vi "Main_SAIDD_1while.vi"() -> ()   [LabVIEW 2018]
uses:
  <vilib>/myRIO/Common/Instrument Driver Framework/myRIO v1.0/UART/vis/myRIO v1.0 Close UART.vi
  <vilib>/Utility/error.llb/Error Cluster From Error Code.vi
  <vilib>/myRIO/Common/Instrument Driver Framework/myRIO v1.0/PWM/vis/myRIO v1.0 Write PWM.vi
  <vilib>/myRIO/Common/Instrument Driver Framework/myRIO v1.0/DIO/vis/myRIO v1.0 Write DIO.vi
  <vilib>/myRIO/Common/Instrument Driver Framework/Utilities/vis/FPGA Ref Manager.vi
  <vilib>/myRIO/Common/Instrument Driver Framework/myRIO v1.0/myRIO v1.0 Reset FPGA.vi
  <vilib>/myRIO/Common/Instrument Driver Framework/myRIO v1.0/IRQ/vis/myRIO v1.0 IRQ Info FGV.vi
  <vilib>/myRIO/Common/Instrument Driver Framework/myRIO v1.0/IRQ/vis/myRIO v1.0 Timer IRQ Info FGV.vi
  <vilib>/myRIO/Common/Instrument Driver Framework/myRIO v1.0/IRQ/vis/myRIO v1.0 ISR Agent.vi
  <vilib>/myRIO/Instrument Drivers/Onboard IO/DIO/DIO.lvlib
  <vilib>/myRIO/Instrument Drivers/Onboard IO/PWM/PWM.lvlib
  <vilib>/myRIO/Instrument Drivers/Utilities/Utilities.lvlib
panel:
  in  "Filter?":bool=TRUE
  out "RollDetection - Alarm":bool
  in  "Radius":dbl=0.005 format="%#_13g"
  in  "high cutoff freq:":dbl=900.0
  in  "Grounded threshold":dbl=1.7 format="%#_13g"
  in  "Enable Triangle Wobble":bool=TRUE
  in  "Antal iterationer pr. stepper":i32=800
  in  "Stop":bool
  out "Measured current":dbl
  out "Ammeter measurement":dbl(graph)
  out "Duty Cycle":dbl
  out "Mean 200":dbl format="%0.2f"
  out "Battery left (%)":dbl
  in  "Drill - Frequency [Hz]":dbl=200.0
  in  "Stepper frekvens ned":dbl=120.0
  in  "Ingen modstand ned upper threshold":dbl=2750.0
  out "ALL TOP":bool
  out "ALL BOTTOM":bool
  in  "Resistance - Threshold Upper":dbl=3100.0
  in  "Resistance Threshold Lower":dbl=3025.0
  out "Process":T1(ring)
  in  "State":T1(ring)
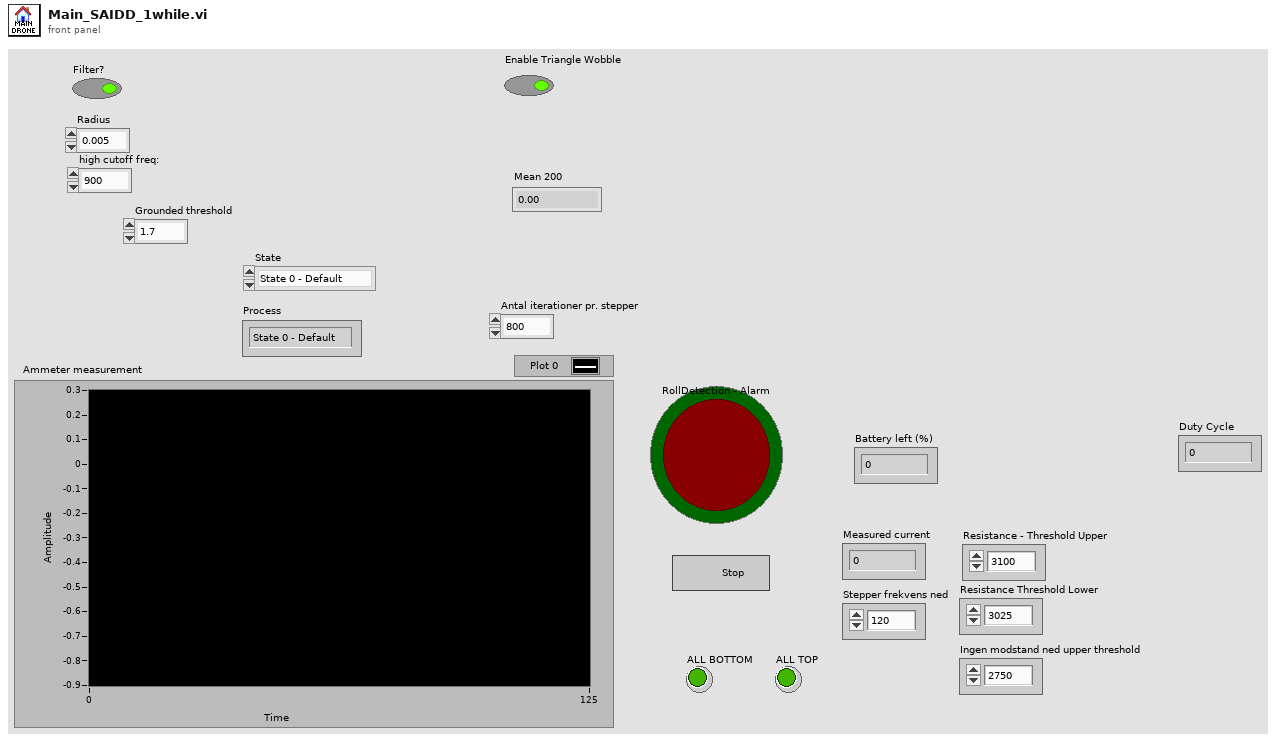
[diagram p1: front panel]
types:
  T1 = enum16{"State 0 - Default", "State 1 - Go down", "State 2 - Go up", "State 3 - Triangle Wobble"}
  T2 = typedef "DIO.lvlib/DIO Reference.ctl" = cluster{"myRIO Reference":T3, "DIO Channels List":T7}
  T3 = typedef "myRIO Generic Hardware Reference.ctl" = cluster{"myRIO Model":T4, "myRIO Hardware Reference":T5}
  T4 = typedef "Hardware Version Enum.ctl" = enum16{"Unknown", "myRIO-1900", "myRIO-1950", "roboRIO", "NI ELVIS RIO CM", "ELVIS III"}
  T5 = typedef "myRIO v1.0 Reference.ctl" = cluster{"Generic FPGA Reference":T6, "Allow multiple opens":bool}
  T6 = typedef "Generic FPGA Reference.ctl" = refnum<k20>
  T7 = typedef "DIO Channels List.ctl" = T8[]
  T8 = typedef "DIO Channels Enum.ctl" = enum16{"Not Connected", "C/DIO0", "C/DIO1", "C/DIO2", "C/DIO3", "C/DIO4", "C/DIO5", "C/DIO6", "C/DIO7", "A/DIO0", "A/DIO1", "A/DIO2", "A/DIO3", "A/DIO4", "A/DIO5", "A/DIO6", "A/DIO7", "A/DIO8", "A/DIO9", "A/DIO10", "A/DIO11", "A/DIO12", "A/DIO13", "A/DIO14", "A/DIO15", "A/DIO16", "A/DIO17", "A/DIO18", "A/DIO19", "B/DIO0", "B/DIO1", "B/DIO2", "B/DIO3", "B/DIO4", "B/DIO5", "B/DIO6", "B/DIO7", "B/DIO8", "B/DIO9", "B/DIO10", "B/DIO11", "B/DIO12", "B/DIO13", "B/DIO14", "B/DIO15", "B/DIO16", "B/DIO17", "B/DIO18", "B/DIO19", "LED0", "LED1", "LED2", "LED3", "Button0", "DIO/DIO0", "DIO/DIO1", "DIO/DIO2", "DIO/DIO3", "DIO/DIO4", "DIO/DIO5", "DIO/DIO6", "DIO/DIO7", "DIO/DIO8", "DIO/DIO9", "SPI/CS0", "SPI/CS1", "SPI/CS2", "SPI/CS3", "LED RADIO (Green)", "LED RADIO (Red)", "LED COMM (Green)", "LED COMM (Red)", "LED MODE (Green)", "LED MODE (Red)"}
  T9 = typedef "PWM.lvlib/PWM Reference.ctl" = cluster{"myRIO Reference":T3, "PWM Channels Enum":T10, "PWM Configuration":T11}
  T10 = typedef "PWM Channels Enum.ctl" = enum16{"Not Connected", "C/PWM0", "C/PWM1", "A/PWM0", "A/PWM1", "A/PWM2", "A/PWM3", "A/PWM4", "A/PWM5", "A/PWM6", "A/PWM7", "A/PWM8", "A/PWM9", "A/PWM10", "A/PWM11", "A/PWM12", "A/PWM13", "A/PWM14", "A/PWM15", "A/PWM16", "A/PWM17", "A/PWM18", "A/PWM19", "B/PWM0", "B/PWM1", "B/PWM2", "B/PWM3", "B/PWM4", "B/PWM5", "B/PWM6", "B/PWM7", "B/PWM8", "B/PWM9", "B/PWM10", "B/PWM11", "B/PWM12", "B/PWM13", "B/PWM14", "B/PWM15", "B/PWM16", "B/PWM17", "B/PWM18", "B/PWM19", "PWM/PWM0", "PWM/PWM1", "PWM/PWM2", "PWM/PWM3", "PWM/PWM4", "PWM/PWM5", "PWM/PWM6", "PWM/PWM7", "PWM/PWM8", "PWM/PWM9"}
  T11 = typedef "PWM.lvlib/PWM Configuration.ctl" = cluster{"Frequency":dbl, "Duty Cycle":dbl}
  T12 = typedef "Accelerometer.lvlib/Accelerometer Reference.ctl" = cluster{"myRIO Reference":T3, "Accelerometer Channels List":T13, "LSB Weight":dbl}
  T13 = typedef "Accelerometer Channels List.ctl" = T14[]
  T14 = typedef "Accelerometer Channels Enum.ctl" = enum16{"Not Connected", "X-Axis", "Y-Axis", "Z-Axis"}
  T15 = typedef "AI.lvlib/AI Reference.ctl" = cluster{"myRIO Reference":T3, "AI Channels List":T16, "AI Scaling Constants List":T18}
  T16 = typedef "AI Channels List.ctl" = T17[]
  T17 = typedef "AI Channels Enum.ctl" = enum16{"Not Connected", "AudioIn/Left", "AudioIn/Right", "C/AI0", "C/AI1", "A/AI0", "A/AI1", "A/AI2", "A/AI3", "A/AI4", "A/AI5", "A/AI6", "A/AI7", "B/AI0", "B/AI1", "B/AI2", "B/AI3", "B/AI4", "B/AI5", "B/AI6", "B/AI7", "AI/AI0", "AI/AI1", "AI/AI2", "AI/AI3", "A/AI0 (DIFF)", "A/AI1 (DIFF)", "A/AI2 (DIFF)", "A/AI3 (DIFF)", "B/AI0 (DIFF)", "B/AI1 (DIFF)", "B/AI2 (DIFF)", "B/AI3 (DIFF)"}
  T18 = typedef "Analog Scaling Constants List.ctl" = T19[]
  T19 = typedef "Analog Scaling Constants.ctl" = cluster{"LSB Weight (Volts)":dbl, "Offset (Volts)":dbl, "Signed?":bool}
  T20 = typedef "SPI.lvlib/SPI Reference.ctl" = cluster{"myRIO Reference":T3, "SPI Channels Enum":T21, "SPI Configuration":T22}
  T21 = typedef "SPI Channels Enum.ctl" = enum16{"Not Connected", "A/SPI", "B/SPI", "SPI/SPI"}
  T22 = typedef "SPI.lvlib/SPI Configuration.ctl" = cluster{"Frequency [Hz]":dbl, "Clock Phase":T23, "Clock Polarity":T24, "Data Direction":T25, "Frame Length":T26}
  T23 = typedef "SPI Clock Phase.ctl" = enum8{"Leading", "Trailing"}
  T24 = typedef "SPI Clock Polarity.ctl" = enum8{"Low", "High"}
  T25 = typedef "SPI Data Direction.ctl" = enum8{"Most significant bit first", "Least significant bit first"}
  T26 = typedef "SPI Frame Length.ctl" = u8
  T27 = cluster{"B/DIO0 - Stepper Direction":T2, "B/DIO1 - Stepper1 Enable":T2, "B/DIO2 - Stepper2 Enable":T2, "B/DIO3 - Stepper3 Enable":T2, "B/DIO4 - Endstop Stepper1 Top":T2, "B/DIO11 - Endstop Stepper1 Bund":T2, "B/DIO12 - Endstop Stepper2 Top":T2, "B/DIO13 - Endstop Stepper2 Bund":T2, "B/DIO14 - Endstop Stepper3 Top":T2, "B/DIO15 - Endstop Stepper3 Bund":T2, "Deleted - A/DIO0 - Cooler":T2, "A/DIO1 - Beacon drop (dio1)":T2, "A/DIO2 - Beacon drop (dio0)":T2, "A/DIO3 - QuickRelease (dio1)":T2, "A/DIO4 - QuickRelease (dio0)":T2, "Deleted - A/DIO11 - LiDAR SPI CS":T2, "B/PWM0 - Stepper":T9, "B/PWM1 - Drill":T9, "Deleted - A/PWM0 - Servo_Roll":T9, "Deleted - A/PWM1 - Servo_Yaw":T9, "Acc. X-axis":T12, "Acc. Y-axis":T12, "B/AI0 - Drone Grounded S1 - F3":T15, "A/AI0 - QuickRelease S4 - F4":T15, "B/AI2 - Beacon Drop S5 - F5":T15, "B/AI3 - Begin drilling S3 - F6":T15, "B/AI1 - Gimbal Seach S8 - F8":T15, "Deleted - A/AI1 - Beacon Wiper":T15, "A/AI2 - QuickRelease Wiper":T15, "A/AI3 - Drill Current":T15, "Deleted - A/SPI - LiDAR":T20, "B/UART - XBee":refnum<visa-resource-name>, "Deleted - A/UART - A3 GPS":refnum<visa-resource-name>, "RIO Flashing LEDs":T2}
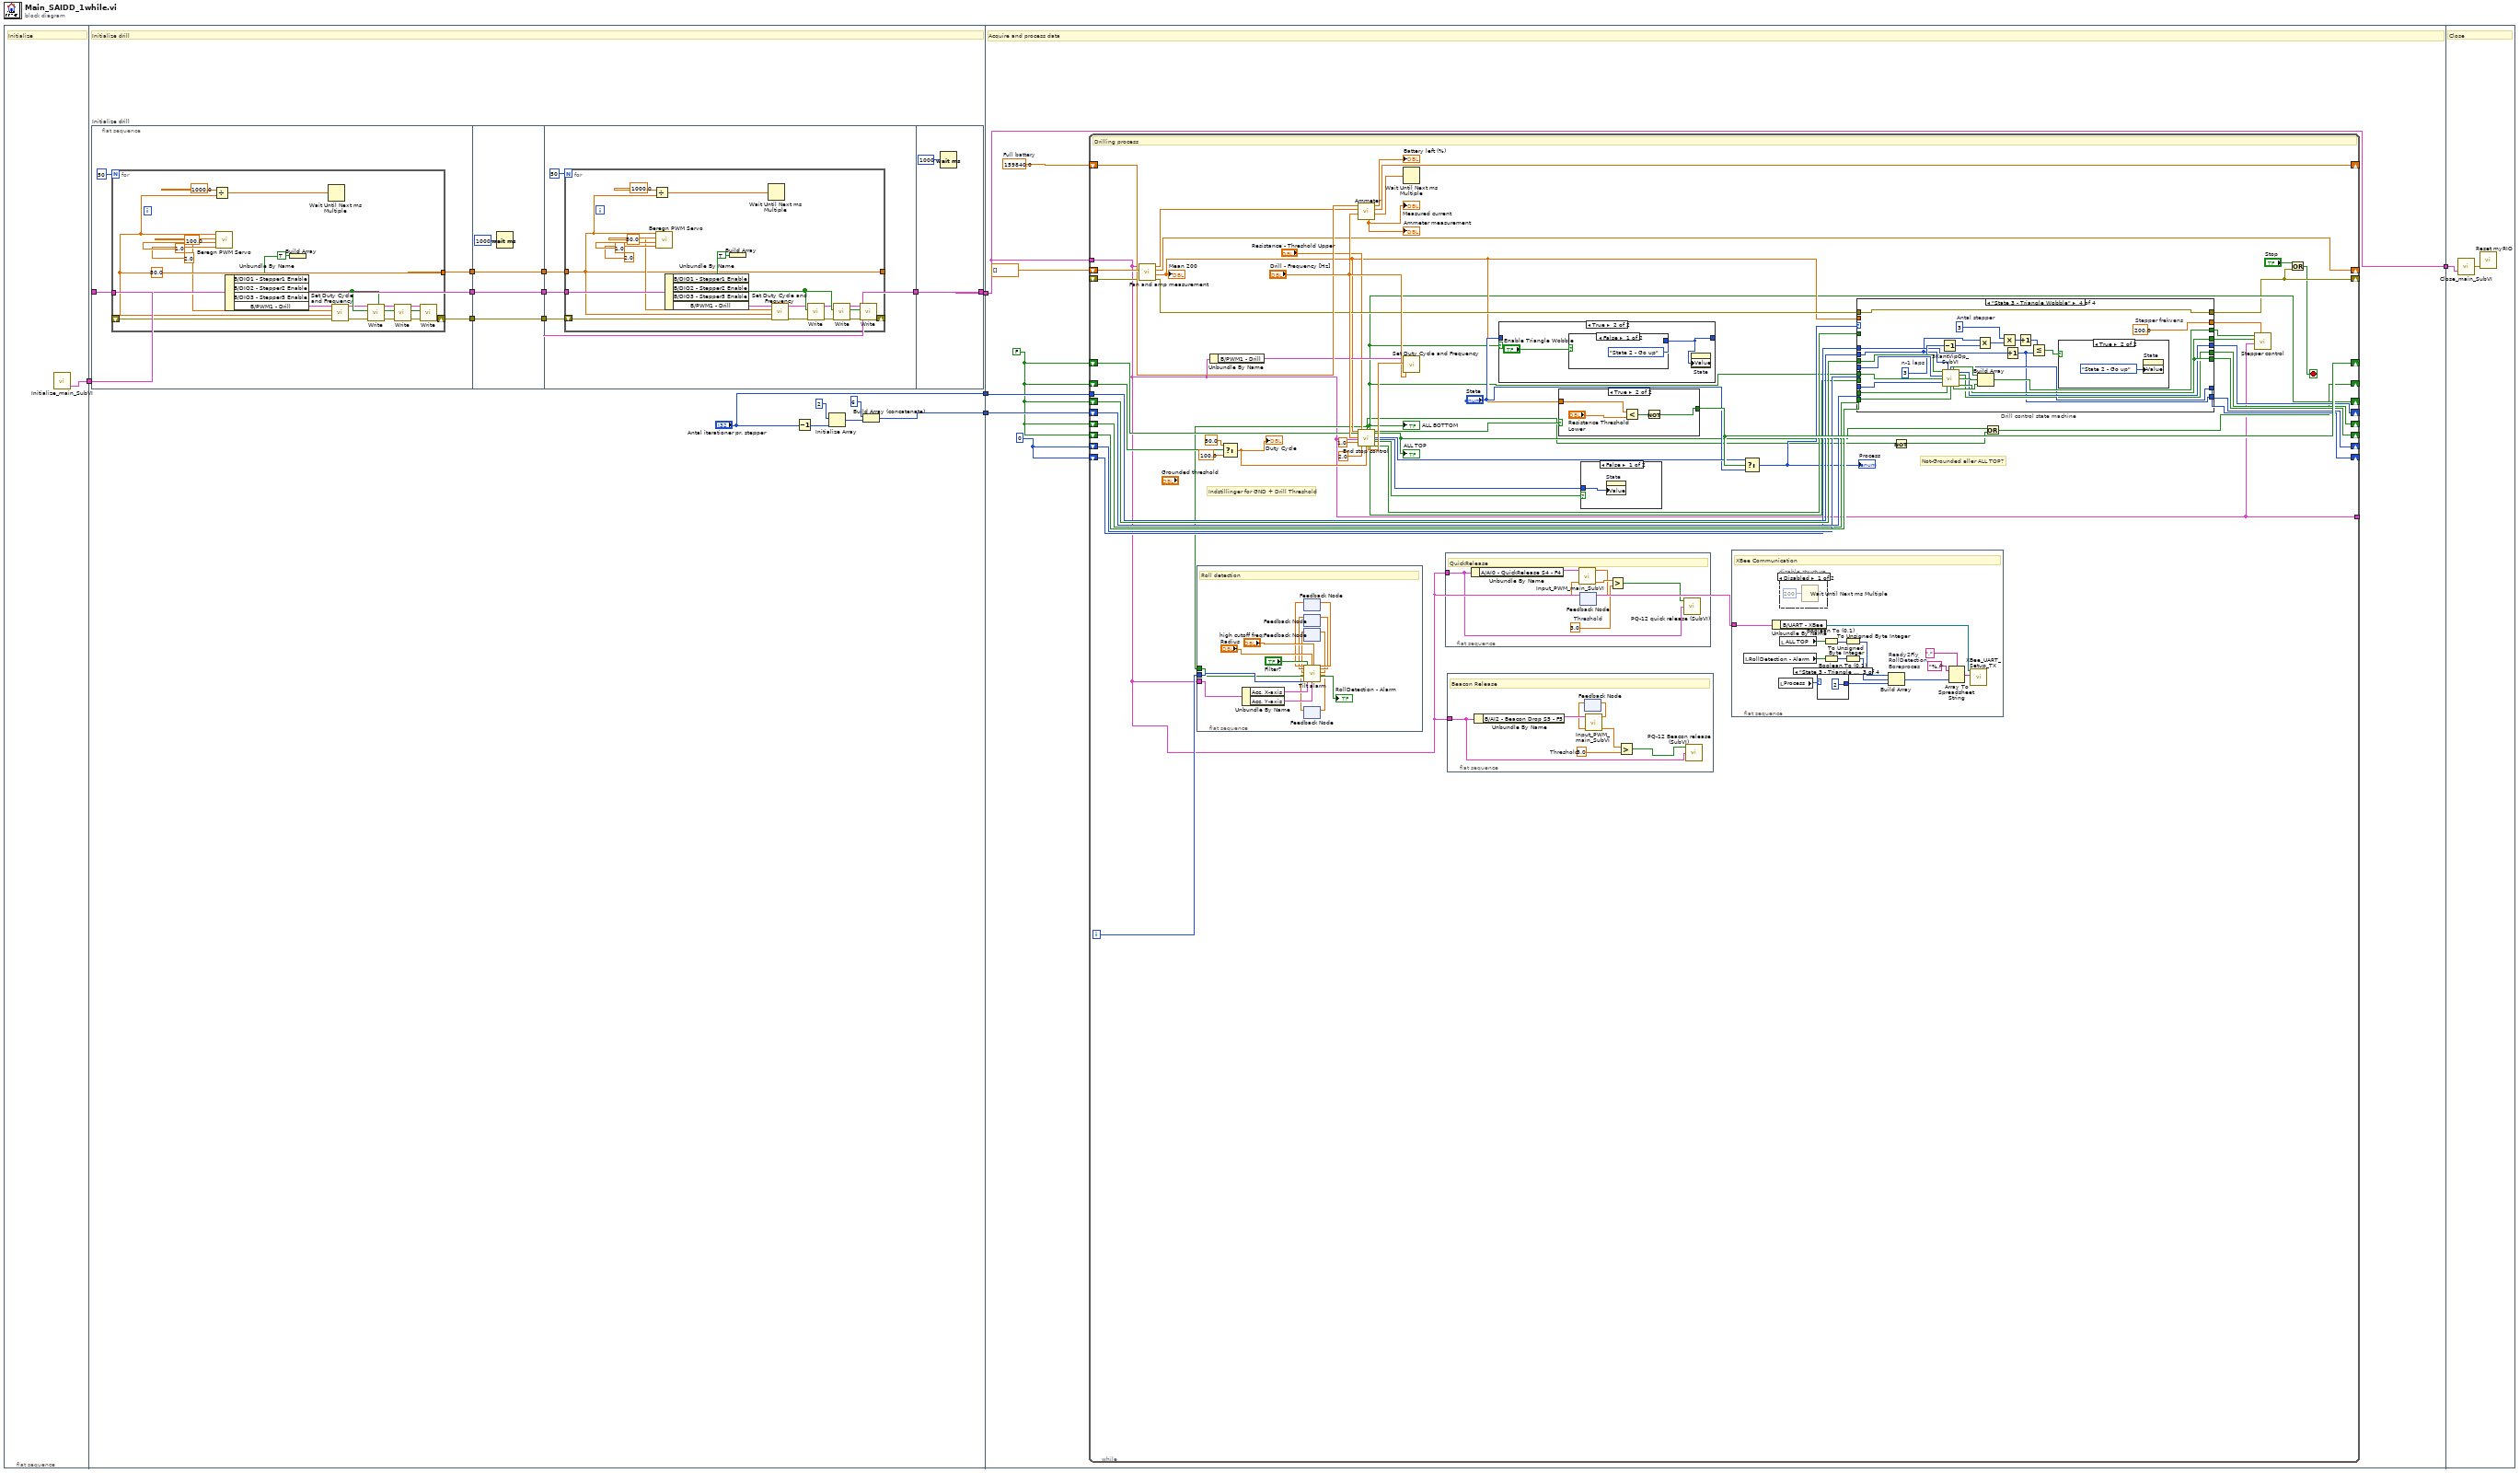
[diagram p0: block diagram]
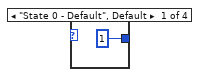
[diagram p3: hidden frame]
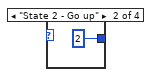
[diagram p4: hidden frame]
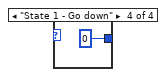
[diagram p5: hidden frame]
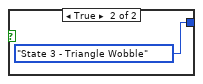
[diagram p8: hidden frame]
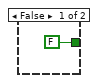
[diagram p9: hidden frame]
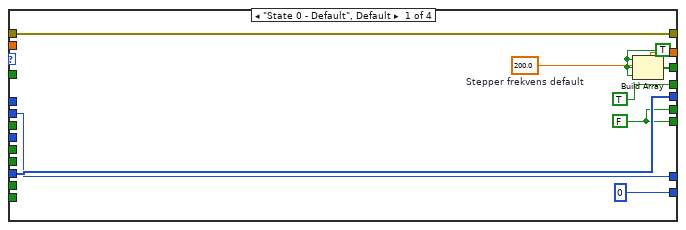
[diagram p10: hidden frame]
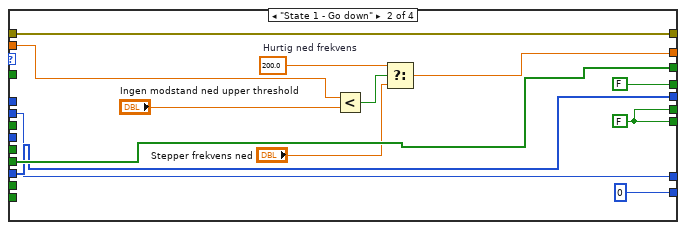
[diagram p11: hidden frame]
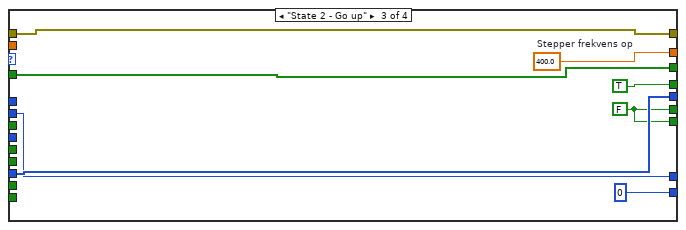
[diagram p12: hidden frame]
diagram:
  n1 = flat-sequence {
    tunnel: [w6] -> w4
    tunnel: w4 -> [w21]
    tunnel: [w18] -> w3
    tunnel: ["Antal iterationer pr. stepper"] -> w2
    tunnel: [w12] -> w1
    tunnel: w3 -> [w74]
    tunnel: [w74] -> w5
    tunnel: w2 -> [w77]
    tunnel: w1 -> [w76]
    tunnel: w5 -> [w256]
    frame #0 {
      # "Initialize"
      n2 = call "Initialize_main_SubVI.vi"() -> ("output cluster"=w6:T27)  [unwired: 2 in, 1 out]
    }
    frame #1 {
      # "Initialize drill"
      n3 = flat-sequence "Initialize drill" {
        tunnel: w21 -> [w25]
        tunnel: [w25] -> w20
        tunnel: [w24] -> w9
        tunnel: [w23] -> w7
        tunnel: w20 -> [w48]
        tunnel: [w48] -> w19
        tunnel: [w46] -> w10
        tunnel: w9 -> [w46]
        tunnel: [w45] -> w8
        tunnel: w7 -> [w45]
        tunnel: w19 -> [w52]
        tunnel: [w52] -> w17
        tunnel: w10 -> [w51]
        tunnel: w8 -> [w50]
        tunnel: [w73] -> w18
        tunnel: w17 -> [w73]
        frame #0 {
          n4 = for {
            N: 50 -> [_]
            tunnel: [w39] -> w24
            shift-right: [w32] -> w23
            shift-left: _ -> [w41]
            tunnel: w25 -> [w37]
            w39 = 50.0 ("Frequency [Hz]")
            n5 = Divide(x=1000.0, y=w39) -> (x/y=w40:dbl)
            n6 = call "Beregn PWM Servo.vi"("Max (ms puls bredde)"=2.0, "Min (ms puls bredde)"=1.0, "Duty Cycle"=100.0, "Frekvens"=w39) -> ("Output Dutycycle til PWM Servo"=w26:dbl)  [unwired: 7 in]
            n7 = Unbundle By Name(w37) -> ("B/DIO1 - Stepper1 Enable"=w27:T2, "B/DIO2 - Stepper2 Enable"=w28:T2, "B/DIO3 - Stepper3 Enable"=w29:T2, "B/PWM1 - Drill"=w31:T9)
            n8 = Build Array(TRUE) -> (w30:bool[])
            n9 = Wait Until Next ms Multiple(millisecond multiple=w40) -> ()  [unwired: 1 out]
            n10 = call <vilib>:"Set Duty Cycle and Frequency.vi"("error in (no error)"=w41, "Frequency [Hz]"=w39, "Duty Cycle"=w26, "PWM Ref In"=w31) -> ("error out"=w35:errorcluster)  [unwired: 5 in, 1 out]
            n11 = call <vilib>:"Write.vi"("error in (no error)"=w35, "Values"=w30, "DIO Ref In"=w29) -> ("error out"=w34:errorcluster)  [unwired: 6 in, 1 out]
            n12 = call <vilib>:"Write.vi"("error in (no error)"=w34, "Values"=w30, "DIO Ref In"=w28) -> ("error out"=w33:errorcluster)  [unwired: 6 in, 1 out]
            n13 = call <vilib>:"Write.vi"("error in (no error)"=w33, "Values"=w30, "DIO Ref In"=w27) -> ("error out"=w32:errorcluster)  [unwired: 6 in, 1 out]
          }
        }
        frame #1 {
          n14 = Wait (ms)(milliseconds to wait=u32 1000) -> ()  [unwired: 1 out]
        }
        frame #2 {
          n15 = for {
            N: 50 -> [_]
            tunnel: [w53] -> _
            shift-right: [w60] -> _
            shift-left: w50 -> [w68]
            tunnel: w52 -> [w65]
            tunnel: w51 -> [w53]
            n16 = Divide(x=1000.0, y=w53) -> (x/y=w67:dbl)
            n17 = call "Beregn PWM Servo.vi"("Max (ms puls bredde)"=2.0, "Min (ms puls bredde)"=1.0, "Duty Cycle"=50.0, "Frekvens"=w53) -> ("Output Dutycycle til PWM Servo"=w54:dbl)  [unwired: 7 in]
            n18 = Unbundle By Name(w65) -> ("B/DIO1 - Stepper1 Enable"=w55:T2, "B/DIO2 - Stepper2 Enable"=w56:T2, "B/DIO3 - Stepper3 Enable"=w57:T2, "B/PWM1 - Drill"=w59:T9)
            n19 = Build Array(TRUE) -> (w58:bool[])
            n20 = Wait Until Next ms Multiple(millisecond multiple=w67) -> ()  [unwired: 1 out]
            n21 = call <vilib>:"Set Duty Cycle and Frequency.vi"("error in (no error)"=w68, "Frequency [Hz]"=w53, "Duty Cycle"=w54, "PWM Ref In"=w59) -> ("error out"=w63:errorcluster)  [unwired: 5 in, 1 out]
            n22 = call <vilib>:"Write.vi"("error in (no error)"=w63, "Values"=w58, "DIO Ref In"=w57) -> ("error out"=w62:errorcluster)  [unwired: 6 in, 1 out]
            n23 = call <vilib>:"Write.vi"("error in (no error)"=w62, "Values"=w58, "DIO Ref In"=w56) -> ("error out"=w61:errorcluster)  [unwired: 6 in, 1 out]
            n24 = call <vilib>:"Write.vi"("error in (no error)"=w61, "Values"=w58, "DIO Ref In"=w55) -> ("error out"=w60:errorcluster)  [unwired: 6 in, 1 out]
          }
        }
        frame #3 {
          n25 = Wait (ms)(milliseconds to wait=u32 1000) -> ()  [unwired: 1 out]
        }
      }
      n26 = Decrement(x="Antal iterationer pr. stepper") -> (x-1=w16:i32)
      n27 = Initialize Array(2, w16) -> (w15:i32[])
      n28 = Build Array (concatenate)(6, w15) -> (w12:i32[])
    }
    frame #2 {
      w78 = 0 ("Loops shift out")
      w75 = FALSE ("t")
      w80 = 159840.0  # Full battery
      # "Acquire and process data"
      n29 = while {
        shift-right: [w89] -> _
        shift-left: _ -> [w121]
        shift-right: [w93] -> _
        shift-left: dbl[] [] -> [w134]
        shift-right: [w130] -> _
        shift-left: w80 -> [w131]
        tunnel: w74 -> [w81]
        tunnel: [w81] -> _
        shift-right: [w123] -> _
        shift-left: w75 -> [w122]
        shift-right: [w86] -> _
        shift-left: w75 -> [w119]
        shift-right: [w117] -> _
        shift-left: w75 -> [w116]
        shift-right: [w115] -> _
        shift-left: w76 -> [w114]
        tunnel: w77 -> [w108]
        shift-right: [w112] -> _
        shift-left: w78 -> [w113]
        shift-right: [w111] -> _
        shift-left: w75 -> [w110]
        shift-right: [w91] -> _
        shift-left: w75 -> [w109]
        shift-right: [w106] -> _
        shift-left: w78 -> [w107]
        i -> [w83]
        stop <- w84 stop-if-true
        # "Not-Grounded eller ALL TOP?"
        # "Indstillinger for GND + Drill Threshold"
        # "Drilling process"
        n30 = call "Fan and amp measurement.vi"("error in (no error)"=w121, "Array in"=w134, "output cluster"=w81) -> ("error out"=w127:errorcluster, "Mean out"=w92:dbl, "Array out"=w93:dbl[], "dbl Scaled Value"=w125:dbl)  [unwired: 5 in]
        "Mean 200" <- w92
        n31 = flat-sequence {
          tunnel: w83 -> [w186]
          tunnel: w82 -> [w184]
          tunnel: w81 -> [w178]
          frame #0 {
            # "Roll detection"
            n32 = Unbundle By Name(w178) -> ("Acc. X-axis"=w182:T12, "Acc. Y-axis"=w183:T12)
            n33 = feedback #1() -> (w176:dbl[])  [unwired: 1 in]
            n34 = feedback #2() -> (w174:dbl[])  [unwired: 1 in]
            n35 = feedback #3() -> (w172:dbl)  [unwired: 1 in]
            n36 = feedback #4() -> (w170:dbl)  [unwired: 1 in]
            n37 = call "Tilt alarm.vi"("X-Array-Shift-in"=w176, "Y-Array-Shift-in"=w174, "X-Stored-Shift-in"=w172, "Y-Stored-Shift-in"=w170, "Grounded?"=w184, "Iterations"=w186, "Filter?"="Filter?", "Accelerometer Ref X in"=w182, "Radius"="Radius", "Accelerometer Ref Y In"=w183, "high cutoff freq: fh"="high cutoff freq:") -> ("X-Array-Shift-out"=w177:dbl[], "Y-Array-Shift-out"=w175:dbl[], "X-Stored-Shift-out"=w173:dbl, "Y-Stored-Shift-out"=w171:dbl, "Alarm"=→"RollDetection - Alarm":bool)  [unwired: 11 in, 1 out]
            n38 = feedback-in #1(w177) -> ()
            n39 = feedback-in #2(w175) -> ()
            n40 = feedback-in #3(w173) -> ()
            n41 = feedback-in #4(w171) -> ()
          }
        }
        n42 = Unbundle By Name(w81) -> ("B/PWM1 - Drill"=w128:T9)
        n43 = Select(t=50.0, s=w119, f=100.0 ("upper limit")) -> (s? t:f=w90:dbl)
        "Duty Cycle" <- w90
        n44 = call "Ammeter.vi"("Bor - Frequency [Hz]"="Drill - Frequency [Hz]", "Måling ammeter"=w125, "Sum batteri shift in"=w131) -> ("Wait ud"=w124:dbl, "Sum batteri shift ud"=w130:dbl, "Batteri tilbage (%)"=→"Battery left (%)":dbl, "Målt ampere"=→"Measured current" →"Ammeter measurement":dbl)  [unwired: 5 in]
        n45 = call "End stop control.vi"("Threshold Lower"=w92, "t"=w122, "Bor - Frequency [Hz]"="Drill - Frequency [Hz]", "output cluster"=w81, "Min (ms puls bredde)"=1.0, "Threshold Upper"="Resistance - Threshold Upper", "Max (ms puls bredde)"=2.0, "Bor - Duty Cycle"=w90) -> ("Grounded?"=w82:bool, "Output Dutycycle \nPWM"=w133:dbl, "ALL BOTTOM"=w91:bool, "Bottom Array"=w103:bool[], "Boolean 2"=w100:bool, "ALL TOP"=w87:bool, "Enum 2"=w99:T1, "Enum"=w96:T1, "Boolean"=w97:bool, "Top Array"=w102:bool[])  [unwired: 8 in, 2 out]
        "ALL TOP" <- w87
        "ALL BOTTOM" <- w91
        n46 = Wait Until Next ms Multiple(millisecond multiple=w124) -> ()  [unwired: 1 out]
        n47 = call <vilib>:"Set Duty Cycle and Frequency.vi"("Frequency [Hz]"="Drill - Frequency [Hz]", "Duty Cycle"=w133, "PWM Ref In"=w128) -> ()  [unwired: 6 in, 2 out]
        n48 = flat-sequence {
          tunnel: w81 -> [w166]
          frame #0 {
            w167 = 3.0  # Threshold
            # "QuickRelease"
            n49 = Unbundle By Name(w166) -> ("A/AI0 - QuickRelease S4 - F4"=w169:T15)
            n50 = feedback #5() -> (w164:dbl[])  [unwired: 1 in]
            n51 = call "Input_PWM_main_SubVI.vi"("Shift in"=w164, "AI Ref In"=w169) -> ("Value out"=w168:dbl, "Shift out"=w165:dbl[])  [unwired: 1 in, 1 out]
            n52 = feedback-in #5(w165) -> ()
            n53 = Greater?(x=w168, y=w167) -> (0:w163:bool)
            n54 = call "PQ-12 quick release (SubVI).vi"("output cluster"=w166, "Extend / Retract [F/T]"=w163) -> ()  [unwired: 1 in, 1 out]
          }
        }
        n55 = flat-sequence {
          tunnel: w81 -> [w160]
          frame #0 {
            w162 = 3.0  # Threshold
            # "Beacon Release"
            n56 = Unbundle By Name(w160) -> ("B/AI2 - Beacon Drop S5 - F5"=w159:T15)
            n57 = feedback #6() -> (w157:dbl[])  [unwired: 1 in]
            n58 = call "Input_PWM_main_SubVI.vi"("Shift in"=w157, "AI Ref In"=w159) -> ("Value out"=w161:dbl, "Shift out"=w158:dbl[])  [unwired: 1 in, 1 out]
            n59 = feedback-in #6(w158) -> ()
            n60 = Greater?(x=w161, y=w162) -> (0:w156:bool)
            n61 = call "PQ-12 Beacon release (SubVI).vi"("output cluster"=w160, "Extend / Retract [T/F]"=w156) -> ()  [unwired: 1 in, 1 out]
          }
        }
        n62 = case shown="True" w91 {
          tunnel: [w188 w189] -> _
          tunnel: "State" -> [w188 _]
          frame False {
          }
          frame True {
            n63 = case shown="False" "Enable Triangle Wobble" {
              tunnel: [T1."State 2 - Go up" ("Enum") T1."State 3 - Triangle Wobble" ("Enum")] -> w189
              frame False {
              }
              frame True {
              }
            }
            n64 = property on="State" class="Enum (strict)"("Value"=w189) -> ()  [unwired: 2 in, 2 out]
          }
        }
        n65 = case shown="True" w100 {
          tunnel: [FALSE w194] -> w123
          tunnel: w92 -> [_ w196]
          frame False {
          }
          frame True {
            n66 = Less?(x=w196, y="Resistance Threshold Lower") -> (x < y?=w195:bool)
            n67 = Not(x=w195) -> (.not. x?=w194:bool)
          }
        }
        n68 = case shown="False" w97 {
          tunnel: w96 -> [w187 _]
          frame False {
            n69 = property on="State" class="Enum (strict)"("Value"=w187) -> ()  [unwired: 2 in, 2 out]
          }
          frame True {
          }
        }
        n70 = flat-sequence {
          tunnel: w81 -> [w150]
          frame #0 {
            # "XBee Communication"
            n71 = local read "RollDetection - Alarm"() -> (w137:bool)
            n72 = Unbundle By Name(w150) -> ("B/UART - XBee"=w149:refnum<visa-resource-name>)
            n73 = local read "Process"() -> (w144:T1)
            n74 = disable-structure shown="Disabled" {
              frame Disabled {
                n75 = Wait Until Next ms Multiple(millisecond multiple=u32 200) -> ()  [unwired: 1 out]
              }
              frame Enabled {
              }
            }
            n76 = local read "ALL TOP"() -> (w142:bool)
            n77 = case shown="\"State 3 - Triangle Wobble\"" w144 {
              tunnel: [u8 1 u8 2 u8 2 u8 0] -> w143
              frame "State 0 - Default", Default {
              }
              frame "State 2 - Go up" {
              }
              frame "State 3 - Triangle Wobble" {
              }
              frame "State 1 - Go down" {
              }
            }
            n78 = Boolean To (0,1)(Boolean=w142) -> (0, 1=w141:i16)
            n79 = Boolean To (0,1)(Boolean=w137) -> (0, 1=w139:i16)
            n80 = To Unsigned Byte Integer(number=w141) -> (unsigned 8bit integer=w140:u8)
            n81 = To Unsigned Byte Integer(number=w139) -> (unsigned 8bit integer=w138:u8)
            n82 = Build Array "Ready2Fly\nRollDetection\nBoreproces"(w140, w138, w143) -> (w145:u8[])
            n83 = Array To Spreadsheet String(delimiter (Tab)=",", array=w145, 3:"%.f" ("format string")) -> (spreadsheet string=w148:string)
            n84 = call "XBee_UART_Setup_TX.vi"("Characters to Write"=w148, "VISA resource name in"=w149) -> ()  [unwired: 9 in, 1 out]
          }
        }
        n85 = Select(t=w99, s=w123, f="State") -> (s? t:f=w95:T1)
        "Process" <- w95
        n86 = case "Drill control state machine" shown="\"State 3 - Triangle Wobble\"" w95 {
          tunnel: [w204 w219 w227 w248] -> w94
          tunnel: w103 -> [_ w219 _ _]
          tunnel: w102 -> [_ _ w227 _]
          tunnel: [TRUE FALSE TRUE w247] -> w126
          tunnel: w127 -> [w203 w217 w225 w252]
          tunnel: [w203 w217 w225 w252] -> w89
          tunnel: [w202 w214 w224 w253] -> w120
          tunnel: w92 -> [_ w211 _ _]
          tunnel: [w199 w208 w221 w247] -> w117
          tunnel: w116 -> [_ _ _ w246]
          tunnel: [w201 w210 w223 w245] -> w115
          tunnel: w114 -> [w201 w210 w223 w244]
          tunnel: w108 -> [w200 w209 w222 w234]
          tunnel: w113 -> [_ _ _ w243]
          tunnel: [w200 w209 w222 w242] -> w112
          tunnel: [w199 w208 w221 w241] -> w111
          tunnel: w110 -> [_ _ _ w240]
          tunnel: w109 -> [_ _ _ w239]
          tunnel: w91 -> [_ _ _ w237]
          tunnel: w107 -> [_ _ _ w236]
          tunnel: [0 0 0 w231] -> w106
          frame "State 0 - Default", Default {
            w199 = FALSE
            w202 = 200.0  # Stepper frekvens default
            w205 = TRUE
            n87 = Build Array(w205, w205, w205) -> (w204:bool[])
          }
          frame "State 1 - Go down" {
            w208 = FALSE
            w213 = 200.0  # Hurtig ned frekvens
            n88 = Less?(x=w211, y="Ingen modstand ned upper threshold") -> (x < y?=w216:bool)
            n89 = Select(t=w213, s=w216, f="Stepper frekvens ned") -> (s? t:f=w214:dbl)
          }
          frame "State 2 - Go up" {
            w221 = FALSE
            w224 = 400.0  # Stepper frekvens op
          }
          frame "State 3 - Triangle Wobble" {
            w232 = 3  # Antal stepper
            w238 = 3  # n-1 laps
            w253 = 200.0  # Stepper frekvens
            n90 = Decrement(x=w238) -> (x-1=w235:i32)
            n91 = call "3KantVipOp_SubVI.vi"("Shift 1 in"=w239, "Antal iterationer pr. stepper"=w234, "Loops shift in"=w243, "BUND!"=w237, "Index step array shift in"=w244, "Shift 2 in"=w240, "Shift 3 in"=w246) -> ("Loops shift out"=w242:i32, "Enable 1"=w249:bool, "Index step array shift ud"=w245:i32[], "Shift 2 ud"=w241:bool, "Enable 2"=w250:bool, "Enable 3"=w251:bool, "Direction"=w247:bool)  [unwired: 1 in, 1 out]
            n92 = Multiply(x=w234, y=w235) -> (x*y=w233:i32)
            n93 = Build Array(w249, w250, w251) -> (w248:bool[])
            n94 = Multiply(x=w232, y=w233) -> (x*y=w229:i32)
            n95 = Increment(x=w236) -> (x+1=w231:i32)
            n96 = Increment(x=w229) -> (x+1=w228:i32)
            n97 = Less Or Equal?(x=w228, y=w231) -> (x <= y?=w230:bool)
            n98 = case shown="True" w230 {
              frame False {
              }
              frame True {
                n99 = property on="State" class="Enum (strict)"("Value"=T1."State 2 - Go up" ("Enum")) -> ()  [unwired: 2 in, 2 out]
              }
            }
          }
        }
        n100 = Not(x=w82) -> (.not. x?=w85:bool)
        n101 = Or(x=w87, y=w85) -> (x .or. y?=w86:bool)
        n102 = call "Stepper control.vi"("Stepper frekvens"=w120, "output cluster"=w81, "Direction shift ud"=w126, "Array"=w94) -> ()  [unwired: 7 in, 1 out]
        n103 = Or(x="Stop", y=w89) -> (x .or. y?=w84:bool)
      }
    }
    frame #3 {
      # "Close"
      n104 = call "Close_main_SubVI.vi"("output cluster"=w256) -> ("error out"=w255:errorcluster)  [unwired: 1 in]
      n105 = call <vilib>:"Reset myRIO.vi"("error in (no error)"=w255) -> ()  [unwired: 10 in, 1 out]
    }
  }
